vi "Default Colors.vi"(10 "Number of Entries":i32, 11 "Colors[] in":u32[](array[colorbox])) -> (3 "Colors[] out":u32[](array[colorbox]))   [LabVIEW 2018, in "PieChart.lvclass"]
uses:
  PieChart.lvclass
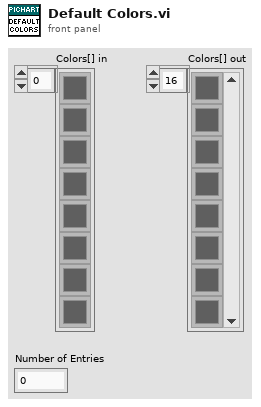
[diagram p1: front panel]
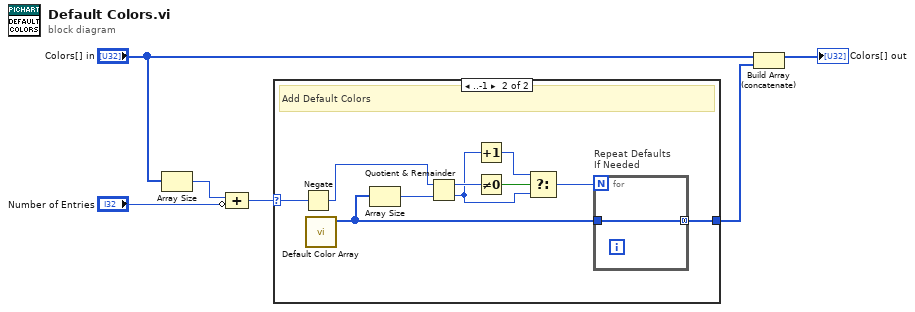
[diagram p0: block diagram]
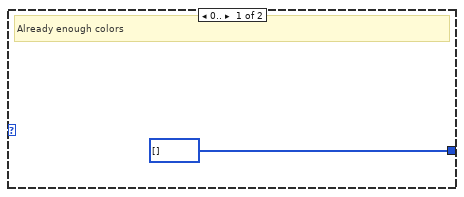
[diagram p2: hidden frame]
diagram:
  n1 = Array Size(array="Colors[] in") -> (size(s)=w6:i32)
  n2 = Compound Arithmetic op=ADD(w6, invert "Number of Entries") -> (w5:i32)
  n3 = case shown="..-1" w5 {
    selector: w5 -> [_ w17]
    tunnel: [u32[] [] ("array") w8] -> w4
    frame 0.. {
      # "Already enough colors"
    }
    frame ..-1 {
      # "Add Default Colors"
      n4 = Negate(x=w17) -> (-x=w15:i32)
      n5 = call "Default Color Array.vi"() -> ("Colors[]"=w9:u32[])  [unwired: 11 in]
      n6 = Array Size(array=w9) -> (size(s)=w16:i32)
      n7 = Quotient & Remainder(x=w15, y=w16) -> (x-y*floor(x/y)=w14:i32, floor(x/y)=w11:i32)
      n8 = Increment(x=w11) -> (x+1=w12:i32)
      n9 = Not Equal To 0?(x=w14) -> (x != 0?=w13:bool)
      n10 = Select(t=w12, s=w13, f=w11) -> (s? t:f=w10:i32)
      n11 = for "Repeat Defaults\nIf Needed" {
        N: w10 -> [_]
        tunnel: w9 -> [w18]
        tunnel: [w18] -> w8 mode=concatenating
      }
    }
  }
  n12 = Build Array (concatenate)("Colors[] in", w4) -> (→"Colors[] out":u32[])
